vi "Template.vi"() -> ()   [LabVIEW 2022 SP3]
panel:
  out "error out":errorcluster
  in  "error in":errorcluster
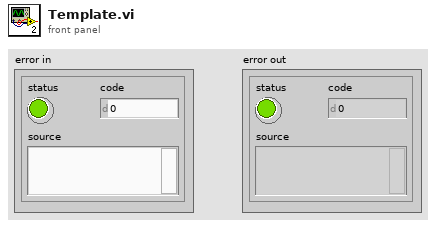
[diagram p1: front panel]
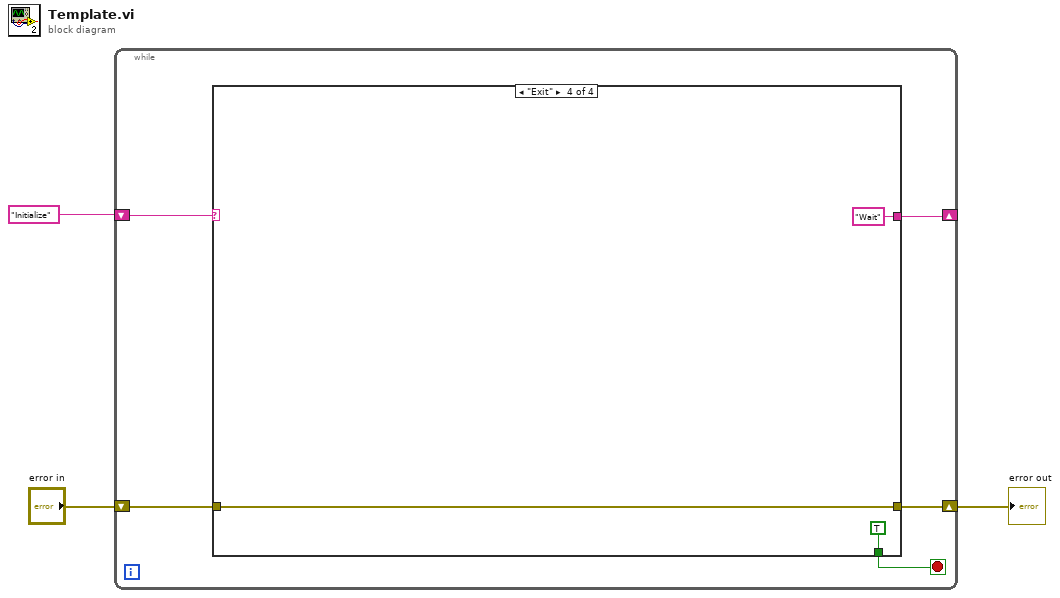
[diagram p0: block diagram]
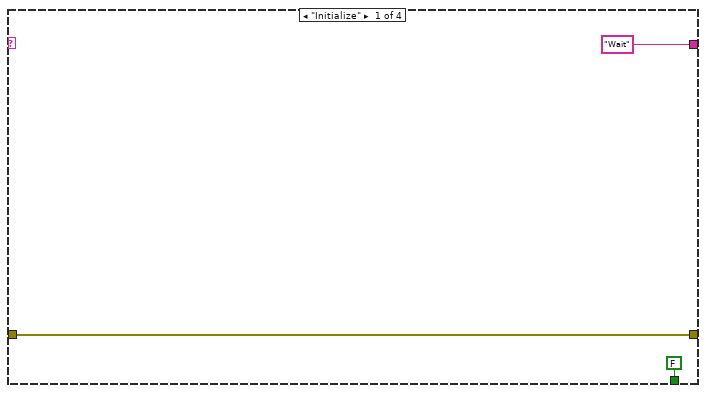
[diagram p2: hidden frame]
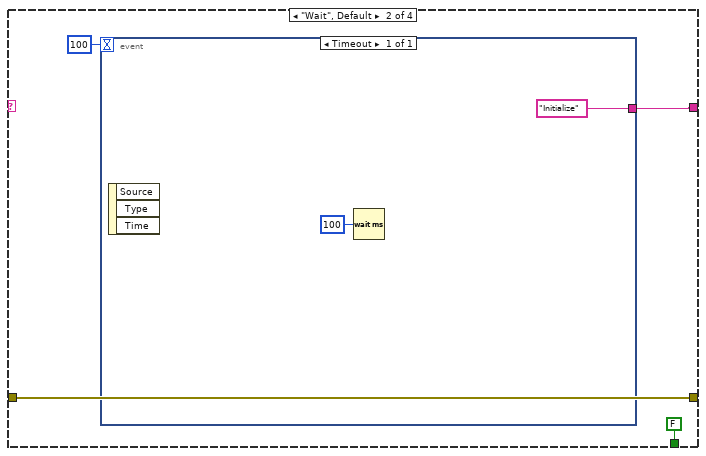
[diagram p3: hidden frame]
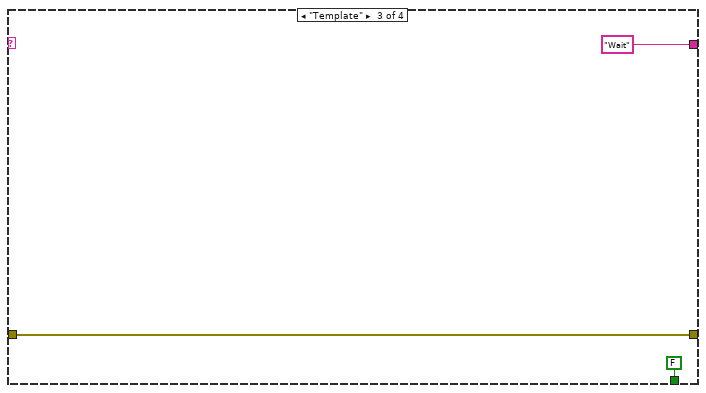
[diagram p4: hidden frame]
diagram:
  n1 = while {
    shift-right: [w7] -> _
    shift-left: "Initialize" -> [w8]
    shift-right: [w4] -> w1
    shift-left: "error in" -> [w5]
    stop <- w6 stop-if-true
    n2 = case shown="\"Exit\"" w8 {
      tunnel: ["Wait" w14 "Wait" "Wait"] -> w7
      tunnel: [FALSE FALSE FALSE TRUE] -> w6
      tunnel: w5 -> [w9 w12 w18 w21]
      tunnel: [w9 w12 w18 w21] -> w4
      frame "Initialize" {
      }
      frame "Wait", Default {
        n3 = event shown="[0] Timeout" {
          selector: _ -> [_]
          dyn-events: _ -> [_]
          timeout: 100 -> [_]
          tunnel: ["Initialize"] -> w14
          event Timeout {
            n4 = event-data() -> ()  [unwired: 1 in, 3 out]
            n5 = Wait (ms)(milliseconds to wait=u32 100) -> ()  [unwired: 1 out]
          }
        }
      }
      frame "Template" {
      }
      frame "Exit" {
      }
    }
  }
  "error out" <- w1
